vi "Half-H Scope.vi"(8 "error in (no error)":errorcluster, 11 "Node Ptr":T2 format="%.0x") -> (0 "error out":errorcluster)   [LabVIEW 2016, in "DCM System Explorer.lvlib"]
uses:
  DCM System Explorer.lvlib
  <vilib>/NI Veristand/Custom Device API/Custom Device Item Ref.ctl
  <vilib>/Powertrain Controls/Device Drivers/DCM/HH/FPGA/Capture Event.ctl
  Shared/DCM Constants and GUIDs.vi
  <vilib>/NI Veristand/Custom Device Tools/Custom Device Utility Library/NI VeriStand - Search for Item by Name.vi
  <vilib>/NI VeriStand/Custom Device API/Custom Device API.lvlib
  DCM Shared.lvlib
  <vilib>/NI Veristand/Custom Device Tools/Custom Device Utility Library/Custom Device Utility Library.lvlib
  <vilib>/Powertrain Controls/Device Drivers/DCM/HH/FPGA/DCM - FPGA - HH.lvlib
panel:
  in  "Capture Event":T1
  in  "Capture Enable":bool
  in  "Capture Length":dbl caption="[s]"
  in  "Header":cluster{"Section Name":string}={"Section Name"="DI Scope Initial Settings"}
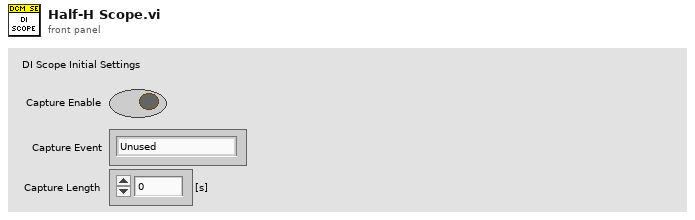
[diagram p1: front panel]
types:
  T1 = typedef "DCM - FPGA - HH.lvlib/Capture Event.ctl" = enum8{"Unused", "HH 1", "HH 2", "HH 3", "HH 4", "HH 5", "HH 6", "HH 7", "HH 8", "HH 9", "HH 10", "HH 11", "HH 12"}
  T2 = typedef "Custom Device API.lvlib/Custom Device Item Ref.ctl" = u64
  T3 = typedef "DCM Shared.lvlib/Channel.ctl" = cluster{"Name":string, "Units":string, "Default":dbl, "Description":string}
  T4 = typedef "Custom Device API.lvlib/Custom Device Channel.ctl" = cluster{"Type":T5, "Units":string, "Default Value":dbl, "Faultable":bool, "Scalable":bool}
  T5 = typedef "Custom Device API.lvlib/Custom Device Channel Type.ctl" = enum16{"Input", "Output"}
  T6 = typedef "Custom Device API.lvlib/Custom Device Commands.ctl" = enum16{"Default", "Item renamed", "Shutdown", "Dynamic button pressed"}
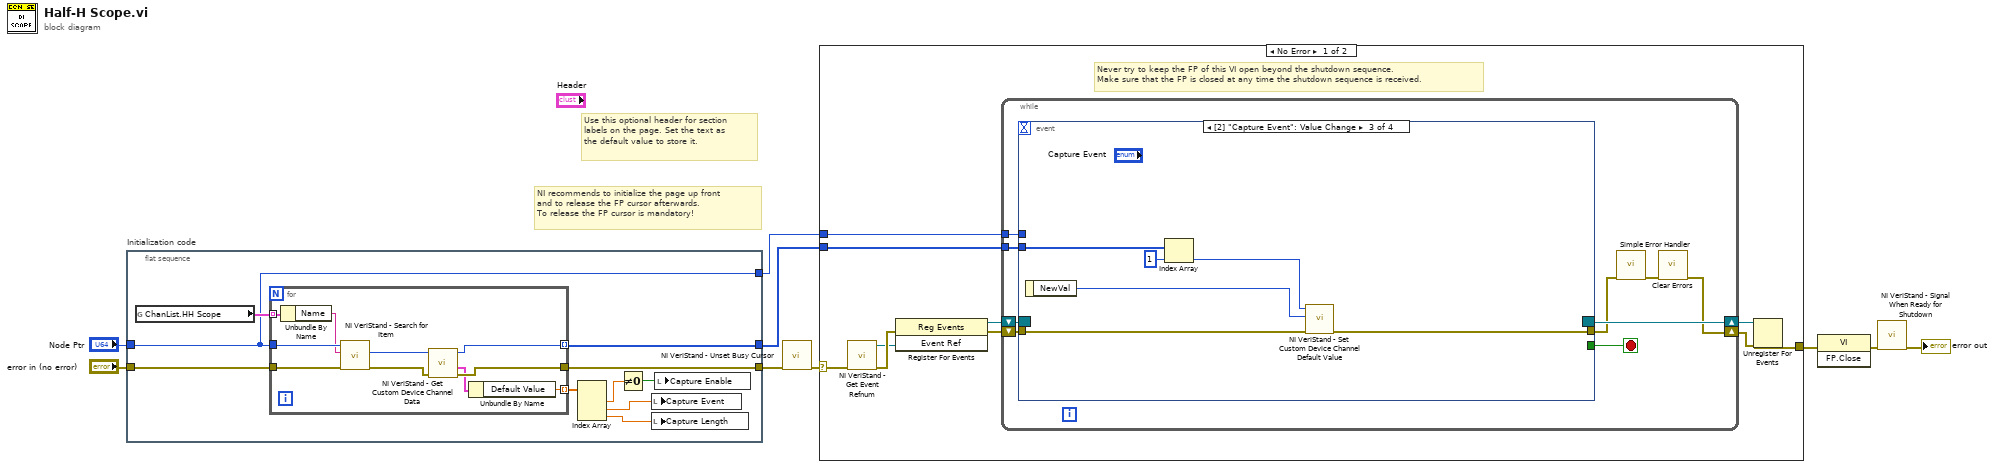
[diagram p0: block diagram]
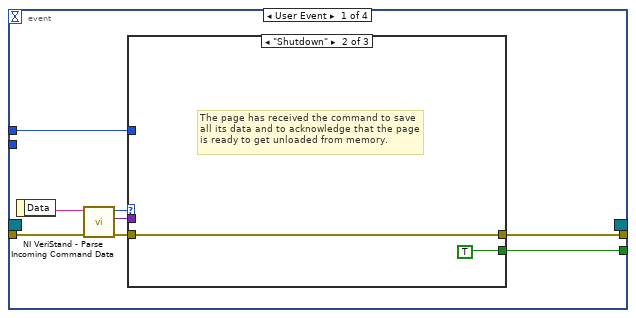
[diagram p2: hidden frame]
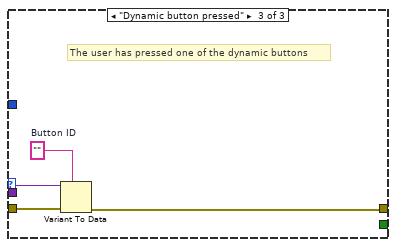
[diagram p4: hidden frame]
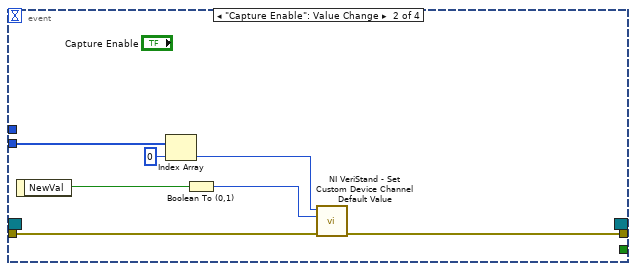
[diagram p5: hidden frame]
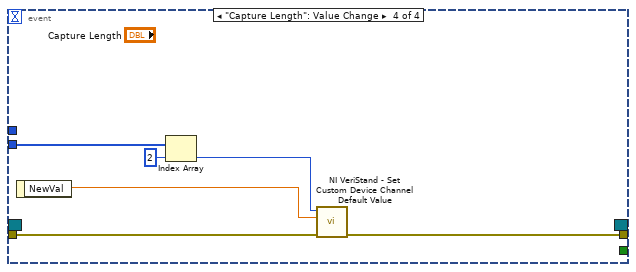
[diagram p6: hidden frame]
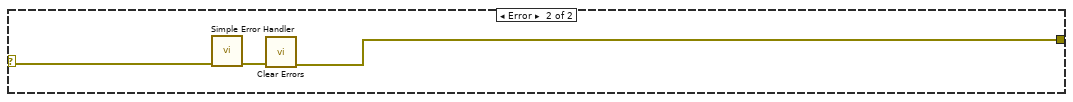
[diagram p7: hidden frame]
diagram:
  # "Use this optional header for section labels on the page. Set the text as the default value to store it."
  # "NI recommends to initialize the page up front\nand to release the FP cursor afterwards.\nTo release the FP cursor is mandatory!"
  n1 = flat-sequence "Initialization code" {
    tunnel: "error in (no error)" -> [w16]
    tunnel: "Node Ptr" -> [w14]
    tunnel: [w19] -> w5
    tunnel: [w15] -> w2
    tunnel: [w14] -> w1
    frame #0 {
      n2 = global read "DCM Constants and GUIDs.vi" "ChanList.HH Scope"() -> (w17:T3[])
      n3 = for {
        tunnel: w14 -> [w29]
        tunnel: w16 -> [w28]
        tunnel: [w20] -> w15 mode=indexing
        tunnel: [w26] -> w19
        tunnel: [w24] -> w18 mode=indexing
        tunnel: w17 -> [w23] mode=indexing
        n4 = Unbundle By Name(w23) -> ("Name"=w22:string)
        n5 = call-poly <vilib>:"NI VeriStand - Search for Item.vi"("error in"=w28, "Item Name"=w22, "Section Ref in"=w29) -> ("error out"=w27:errorcluster, "Item Ref"=w21:T2)  [unwired: 5 in, 2 out]
        n6 = call <vilib>:"NI VeriStand - Get Custom Device Channel Data.vi"("error in (no error)"=w27, "Channel Ref in"=w21) -> ("error out"=w26:errorcluster, "Channel"=w25:T4, "Channel Ref out"=w20:T2)  [unwired: 4 in, 3 out]
        n7 = Unbundle By Name(w25) -> ("Default Value"=w24:dbl)
      }
      n8 = Index Array(array=w18) -> (element #1=w12:dbl, element #2=w10:dbl, element #3=w11:dbl)  [unwired: 3 in]
      n9 = Not Equal To 0?(x=w12) -> (x != 0?=w13:bool)
      n10 = local write "Capture Event"(w10) -> ()
      n11 = local write "Capture Length"(w11) -> ()
      n12 = local write "Capture Enable"(w13) -> ()
    }
  }
  n13 = call <vilib>:"NI VeriStand - Unset Busy Cursor.vi"("error in (no error)"=w5) -> ("error out"=w4:errorcluster)  [unwired: 10 out]
  n14 = case shown="No Error" w4 {
    selector: w4 -> [w31 w85]
    tunnel: [w36 w83] -> w9
    tunnel: w2 -> [w32 _]
    tunnel: w1 -> [w30 _]
    frame No Error {
      # "Never try to keep the FP of this VI open beyond the shutdown sequence.\nMake sure that the FP is closed at any time the shutdown sequence is received."
      n15 = call <vilib>:"NI VeriStand - Get Event Refnum.vi"("error in (no error)"=w31) -> ("error out"=w39:errorcluster, "Event Ref"=w35:refnum<user-event>)  [unwired: 9 out]
      n16 = register-events(error in=w39, w35) -> (reference out=w33:refnum<event-registration>, error out=w34:errorcluster)  [unwired: 1 in]
      n17 = while {
        tunnel: w32 -> [w44]
        shift-right: [w41] -> w37
        shift-left: w34 -> [w47]
        shift-right: [w48] -> w38
        shift-left: w33 -> [w46]
        tunnel: w30 -> [w40]
        stop <- w45 stop-if-true
        n18 = event shown="[2] \"Capture Event\": Value Change" {
          selector: w46 -> [_ _ _ _]
          dyn-events: [_ _ _ _] -> w48
          timeout: _ -> [_ _ _ _]
          tunnel: w47 -> [w56 w68 w74 w80]
          tunnel: [w52 _ _ _] -> w45
          tunnel: [w51 w70 w76 w82] -> w43
          tunnel: w44 -> [_ w67 w73 w79]
          tunnel: w40 -> [w49 _ _ _]
          event User Event {
            n19 = event-data() -> ("Data"=w55:string)  [unwired: 1 out]
            n20 = call <vilib>:"NI VeriStand - Parse Incoming Command Data.vi"("error in (no error)"=w56, "Incoming data"=w55) -> ("error out"=w54:errorcluster, "Outgoing data"=w50:variant, "Action"=w53:T6)  [unwired: 7 out]
            n21 = case shown="\"Shutdown\"" w53 {
              tunnel: w54 -> [w57 w58 w63]
              tunnel: [_ TRUE _] -> w52
              tunnel: [w57 w58 w60] -> w51
              tunnel: w50 -> [_ _ w62]
              tunnel: w49 -> [_ _ _]
              frame "Default", Default {
              }
              frame "Shutdown" {
                # "The page has received the command to save all its data and to acknowledge that the page is ready to get unloaded from memory."
              }
              frame "Dynamic button pressed" {
                w61 = ""  # Button ID
                # "The user has pressed one of the dynamic buttons"
                n22 = Variant To Data(error in=w63, type=w61, Variant=w62) -> (error out=w60:errorcluster)  [unwired: 1 out]
              }
            }
          }
          event "Capture Enable": Value Change {
            n23 = event-data() -> ("NewVal"=w69:bool)  [unwired: 1 out]
            n24 = Index Array(array=w67, index=0) -> (element=w65:T2)
            n25 = Boolean To (0,1)(Boolean=w69) -> (0, 1=w64:i16)
            n26 = call <vilib>:"NI VeriStand - Set Custom Device Channel Default Value.vi"("error in (no error)"=w68, "Default Value"=w64, "Channel Ref in"=w65) -> ("error out"=w70:errorcluster)  [unwired: 7 in, 1 out]
          }
          event Value Change {
            n27 = event-data() -> ("NewVal"=w75:T1)  [unwired: 1 out]
            n28 = Index Array(array=w73, index=1) -> (element=w71:T2)
            n29 = call <vilib>:"NI VeriStand - Set Custom Device Channel Default Value.vi"("error in (no error)"=w74, "Default Value"=w75, "Channel Ref in"=w71) -> ("error out"=w76:errorcluster)  [unwired: 7 in, 1 out]
          }
          event "Capture Length": Value Change {
            n30 = event-data() -> ("NewVal"=w81:dbl)  [unwired: 1 out]
            n31 = Index Array(array=w79, index=2) -> (element=w77:T2)
            n32 = call <vilib>:"NI VeriStand - Set Custom Device Channel Default Value.vi"("error in (no error)"=w80, "Default Value"=w81, "Channel Ref in"=w77) -> ("error out"=w82:errorcluster)  [unwired: 7 in, 1 out]
          }
        }
        n33 = call <vilib>:"Simple Error Handler.vi"("error in (no error)"=w43) -> ("error out"=w42:errorcluster)  [unwired: 1 in, 7 out]
        n34 = call <vilib>:"Clear Errors.vi"("error in (no error)"=w42) -> ("error out"=w41:errorcluster)  [unwired: 1 in, 5 out]
      }
      n35 = Unregister For Events(event registration refnum=w38, error in=w37) -> (error out=w36:errorcluster)
    }
    frame Error {
      n36 = call <vilib>:"Simple Error Handler.vi"("error in (no error)"=w85) -> ("error out"=w84:errorcluster)  [unwired: 1 in, 7 out]
      n37 = call <vilib>:"Clear Errors.vi"("error in (no error)"=w84) -> ("error out"=w83:errorcluster)  [unwired: 1 in, 5 out]
    }
  }
  n38 = invoke class="VI" method="FP.Close"(error in=w9) -> (error out=w8:errorcluster)  [unwired: 2 in, 2 out]
  n39 = call <vilib>:"NI VeriStand - Signal When Ready for Shutdown.vi"("error in (no error)"=w8) -> ("error out"=→"error out":errorcluster)  [unwired: 10 out]
